vi "BATT-VOLT1-ABSOLUTE.vi"(10 "Numeric 4":dbl, 11 "Numeric 5":dbl) -> (3 "Boolean":bool)   [LabVIEW 2016]
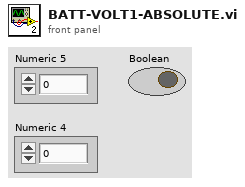
[diagram p1: front panel]
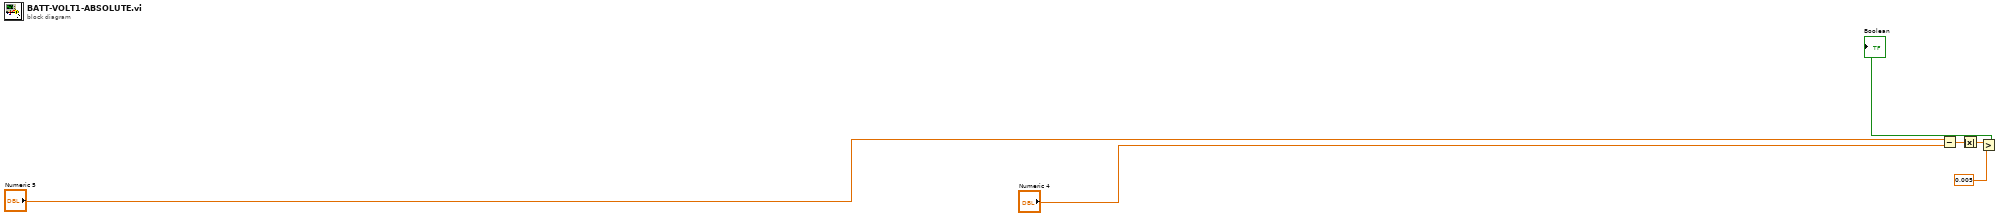
[diagram p0: block diagram]
diagram:
  n1 = Subtract(x="Numeric 5", y="Numeric 4") -> (x-y=w1:dbl)
  n2 = Absolute Value(x=w1) -> (abs(x)=w2:dbl)
  n3 = Greater?(x=w2, y=0.005) -> (0:→"Boolean":bool)
